vi "Acquisition_Main.vi"(8 "error in":errorcluster, 11 "QRD":T1) -> (0 "error out":errorcluster)   [LabVIEW 2025]
uses:
  Controls/Queues-Refs-Data.ctl
  Builds/Queue Wrappers.lvlibp/Q Packet.ctl
  Controls/Local Data_Acquisition.ctl
  Builds/Queue Wrappers.lvlibp
  Data Sources/Instrument A/Instrument A.lvlib
  Data Sources/Instrument B/Instrument B.lvlib
  Data Sources/Instrument C/Instrument C.lvlib
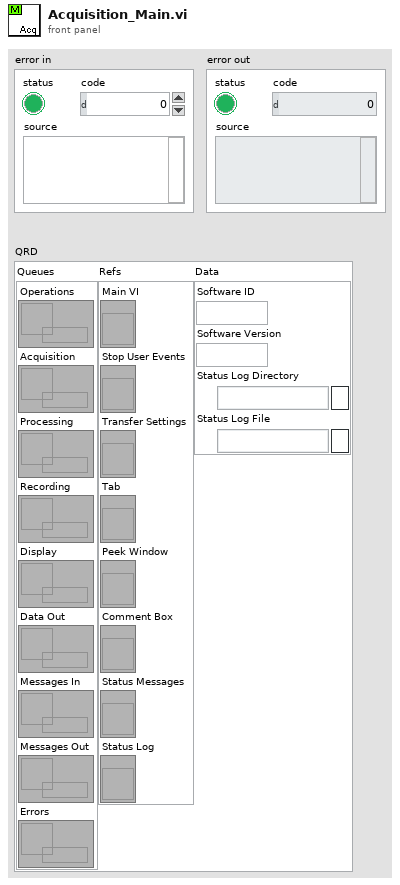
[diagram p1: front panel]
types:
  T1 = typedef "Queues-Refs-Data.ctl" = cluster{"Queues":cluster{"Operations":refnum<queue>, "Acquisition":refnum<queue>, "Processing":refnum<queue>, "Recording":refnum<queue>, "Display":refnum<queue>, "Data Out":refnum<queue>, "Messages In":refnum<queue>, "Messages Out":refnum<queue>, "Errors":refnum<queue>}, "Refs":cluster{"Main VI":refnum<vi>, "Stop User Events":refnum<vi>, "Transfer Settings":refnum<vi>, "Tab":refnum<vi>, "Peek Window":refnum<vi>, "Comment Box":refnum<vi>, "Status Messages":refnum<vi>, "Status Log":refnum<vi>}, "Data":cluster{"Software ID":string, "Software Version":string, "Status Log Directory":path, "Status Log File":path}}
  T2 = typedef "Local Data_Acquisition.ctl" = cluster{"Loop ID":string, "Scan Interval":u32}
  T3 = typedef "Acquisition Packet.ctl" = cluster{"Time Stamp":timestamp, "Raw Data":cluster{"Instrument A":cluster{"Placeholder":string}, "Instrument B":cluster{"Placeholder":string}, "Instrument C":cluster{"Placeholder":string}}, "Derived Data":cluster{"Placeholder":string}}
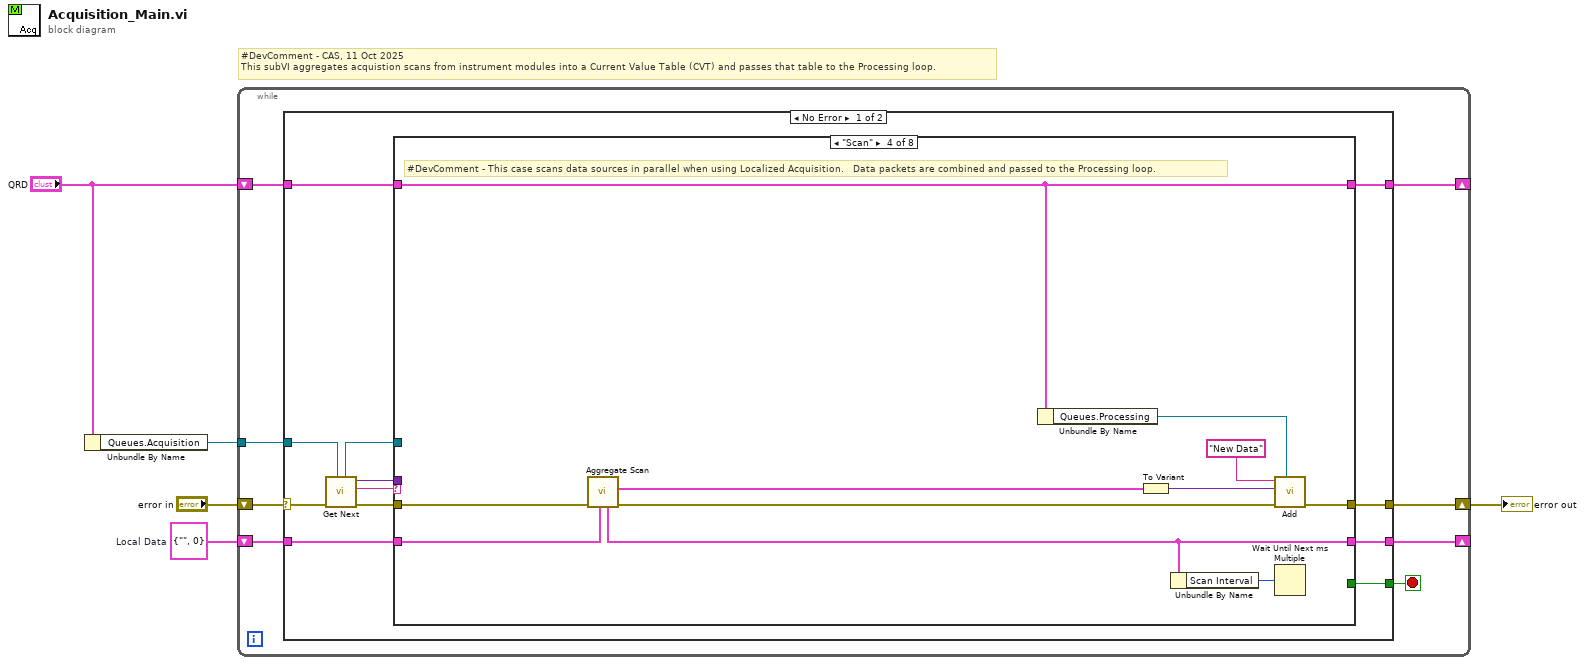
[diagram p0: block diagram]
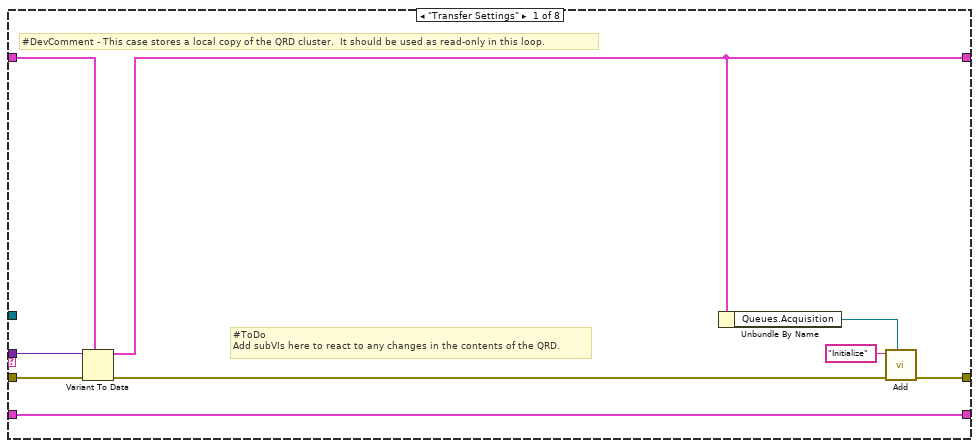
[diagram p2: hidden frame]
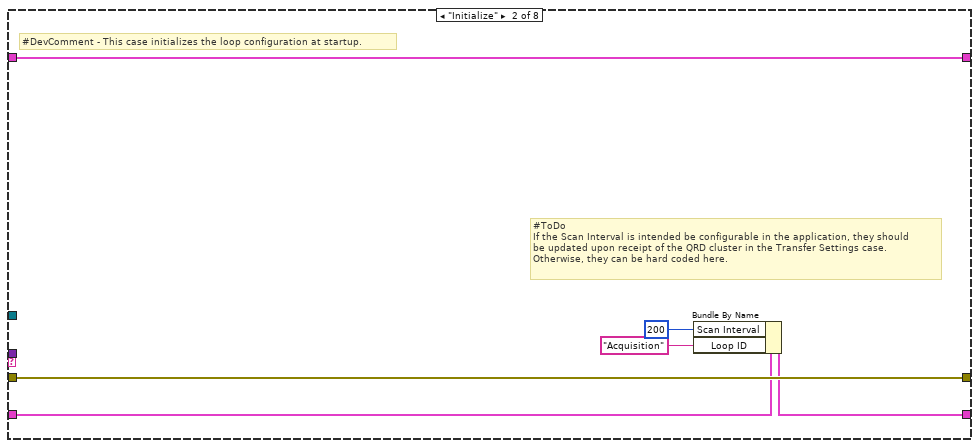
[diagram p3: hidden frame]
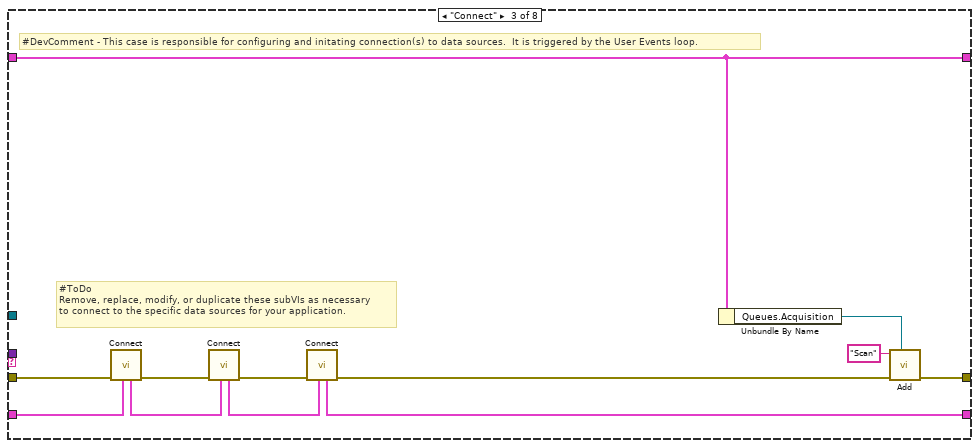
[diagram p4: hidden frame]
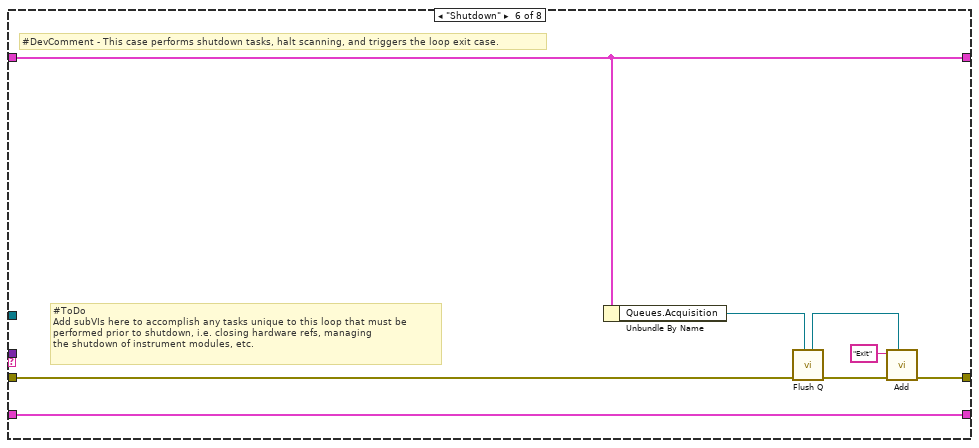
[diagram p6: hidden frame]
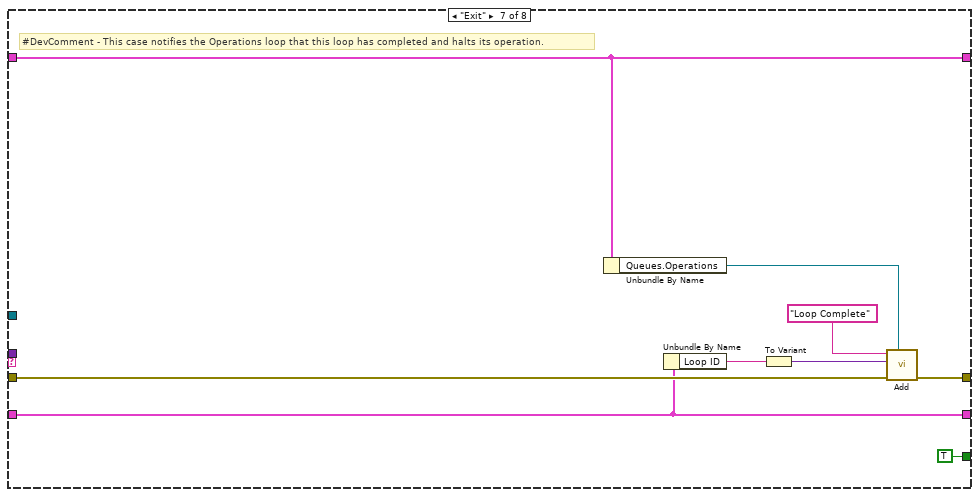
[diagram p7: hidden frame]
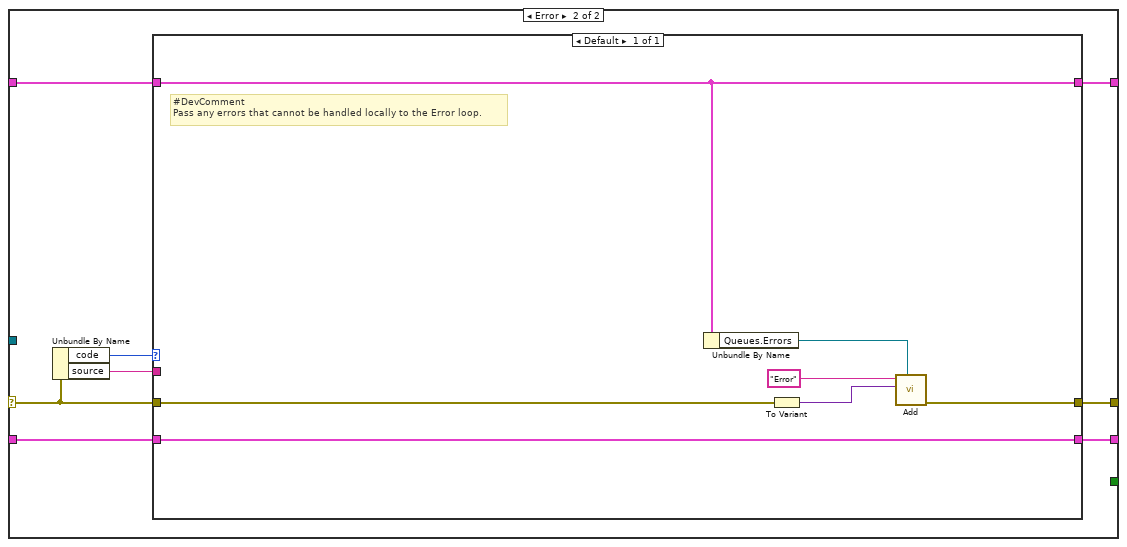
[diagram p9: hidden frame]
diagram:
  w3 = T2 {"Loop ID"="", "Scan Interval"=0}  # Local Data
  # "#DevComment - CAS, 11 Oct 2025\nThis subVI aggregates acquistion scans from instrument modules into a Current Value Table (CVT) and passes that table to the Processing loop."
  n1 = Unbundle By Name("QRD") -> ("Queues.Acquisition"=w1:refnum<queue>)
  n2 = while {
    shift-right: [w12] -> _
    shift-left: "QRD" -> [w13]
    shift-right: [w10] -> w5
    shift-left: "error in" -> [w11]
    tunnel: w1 -> [w9]
    shift-right: [w7] -> _
    shift-left: w3 -> [w8]
    stop <- w6 stop-if-true
    n3 = case shown="No Error" w11 {
      selector: w11 -> [w25 w90]
      tunnel: w13 -> [w22 w87]
      tunnel: [w23 w88] -> w12
      tunnel: [w20 w89] -> w10
      tunnel: w9 -> [w24 _]
      tunnel: w8 -> [w16 w92]
      tunnel: [w15 w91] -> w7
      tunnel: [w14 _] -> w6
      frame No Error {
        n4 = call "Get Next.vi"("Q Ref In"=w24, "error in"=w25) -> ("error out"=w21:errorcluster, "Packet ID"=w17:string, "Payload"=w18:variant, "Q Ref Out"=w19:refnum<queue>)  [unwired: 6 in]
        n5 = case shown="\"Scan\"" w17 {
          tunnel: [w28 w40 w52 w61 w64 w74 w83 w86] -> w23
          tunnel: w22 -> [w31 w40 w52 w61 w64 w74 w83 w86]
          tunnel: w21 -> [w33 w39 w46 w54 w66 w70 w80 w85]
          tunnel: [w29 w39 w50 w60 w66 w72 w82 w85] -> w20
          tunnel: w19 -> [_ _ _ _ _ _ _ _]
          tunnel: w18 -> [w32 _ _ _ _ _ _ _]
          tunnel: w16 -> [w34 w38 w41 w63 w65 w73 w78 w84]
          tunnel: [w34 w37 w42 w55 w65 w73 w78 w84] -> w15
          tunnel: [_ _ _ _ _ _ TRUE _] -> w14
          frame "Transfer Settings" {
            # "#ToDo\nAdd subVIs here to react to any changes in the contents of the QRD."
            # "#DevComment - This case stores a local copy of the QRD cluster.  It should be used as read-only in this loop."
            n6 = Variant To Data(error in=w33, type=w31, Variant=w32) -> (data=w28:T1, error out=w30:errorcluster)
            n7 = Unbundle By Name(w28) -> ("Queues.Acquisition"=w27:refnum<queue>)
            n8 = call "Add.vi"("Q Ref In"=w27, "error in"=w30, "Packet ID"="Initialize") -> ("error out"=w29:errorcluster)  [unwired: 5 in, 3 out]
          }
          frame "Initialize" {
            # "#ToDo\nIf the Scan Interval is intended be configurable in the application, they should\nbe updated upon receipt of the QRD cluster in the Transfer Settings case. \nOtherwise, they can be hard coded here."
            # "#DevComment - This case initializes the loop configuration at startup."
            n9 = Bundle By Name(cluster=w38, "Scan Interval"=u32 200, "Loop ID"="Acquisition") -> (w37:T2)
          }
          frame "Connect" {
            # "#ToDo\nRemove, replace, modify, or duplicate these subVIs as necessary\nto connect to the specific data sources for your application."
            # "#DevComment - This case is responsible for configuring and initating connection(s) to data sources.  It is triggered by the User Events loop."
            n10 = call "Connect.vi"("Local Data"=w41, "error in"=w46) -> ("error out"=w45:errorcluster, "Local Data Out"=w44:T2)  [unwired: 8 in]
            n11 = call "Connect.vi"("Local Data"=w44, "error in"=w45) -> ("error out"=w48:errorcluster, "Local Data Out"=w43:T2)  [unwired: 8 in]
            n12 = call "Connect.vi"("Local Data"=w43, "error in"=w48) -> ("error out"=w47:errorcluster, "Local Data Out"=w42:T2)  [unwired: 8 in]
            n13 = Unbundle By Name(w52) -> ("Queues.Acquisition"=w51:refnum<queue>)
            n14 = call "Add.vi"("Q Ref In"=w51, "error in"=w47, "Packet ID"="Scan") -> ("error out"=w50:errorcluster)  [unwired: 5 in, 3 out]
          }
          frame "Scan" {
            # "#DevComment - This case scans data sources in parallel when using Localized Acquisition.   Data packets are combined and passed to the Processing loop."
            n15 = call "Aggregate Scan.vi"("Local Data"=w63, "error in"=w54) -> ("error out"=w62:errorcluster, "Acquisition Scan"=w53:T3, "Local Data Out"=w55:T2)  [unwired: 7 in]
            n16 = Unbundle By Name(w61) -> ("Queues.Processing"=w59:refnum<queue>)
            n17 = To Variant(anything=w53) -> (Variant=w57:variant)
            n18 = Unbundle By Name(w55) -> ("Scan Interval"=w56:u32)
            n19 = call "Add.vi"("Q Ref In"=w59, "error in"=w62, "Payload"=w57, "Packet ID"="New Data") -> ("error out"=w60:errorcluster)  [unwired: 4 in, 3 out]
            n20 = Wait Until Next ms Multiple(millisecond multiple=w56) -> ()  [unwired: 1 out]
          }
          frame "Disconnect" {
            # "#DevComment - This case commands the shutdown of acquisition modules."
          }
          frame "Shutdown" {
            # "#ToDo\nAdd subVIs here to accomplish any tasks unique to this loop that must be\nperformed prior to shutdown, i.e. closing hardware refs, managing\nthe shutdown of instrument modules, etc."
            # "#DevComment - This case performs shutdown tasks, halt scanning, and triggers the loop exit case."
            n21 = Unbundle By Name(w74) -> ("Queues.Acquisition"=w68:refnum<queue>)
            n22 = call "Flush Q.vi"("Q Ref In"=w68, "error in"=w70) -> ("error out"=w69:errorcluster, "Q Ref Out"=w67:refnum<queue>)  [unwired: 8 in]
            n23 = call "Add.vi"("Q Ref In"=w67, "error in"=w69, "Packet ID"="Exit") -> ("error out"=w72:errorcluster)  [unwired: 5 in, 3 out]
          }
          frame "Exit" {
            # "#DevComment - This case notifies the Operations loop that this loop has completed and halts its operation."
            n24 = Unbundle By Name(w83) -> ("Queues.Operations"=w79:refnum<queue>)
            n25 = Unbundle By Name(w78) -> ("Loop ID"=w77:string)
            n26 = To Variant(anything=w77) -> (Variant=w76:variant)
            n27 = call "Add.vi"("Q Ref In"=w79, "error in"=w80, "Payload"=w76, "Packet ID"="Loop Complete") -> ("error out"=w82:errorcluster)  [unwired: 4 in, 3 out]
          }
          frame Default {
          }
        }
      }
      frame Error {
        n28 = Unbundle By Name(w90) -> ("code"=w94:i32, "source"=w93:string)
        n29 = case shown="Default" w94 {
          tunnel: w93 -> [_]
          tunnel: w92 -> [w101]
          tunnel: [w101] -> w91
          tunnel: w90 -> [w96]
          tunnel: [w98] -> w89
          tunnel: [w97] -> w88
          tunnel: w87 -> [w97]
          frame Default {
            # "#DevComment\nPass any errors that cannot be handled locally to the Error loop."
            n30 = Unbundle By Name(w97) -> ("Queues.Errors"=w99:refnum<queue>)
            n31 = To Variant(anything=w96) -> (Variant=w95:variant)
            n32 = call "Add.vi"("Q Ref In"=w99, "Payload"=w95, "Packet ID"="Error") -> ("error out"=w98:errorcluster)  [unwired: 5 in, 3 out]
          }
        }
      }
    }
  }
  "error out" <- w5
